vi "Actor Core.vi"(8 "error in":errorcluster, 11 "Rotation View in":refnum<class "Rotation View.lvclass">) -> (0 "error out":errorcluster, 3 "Actor out":refnum<class "Actor.lvclass">)   [LabVIEW 2020, in "Rotation View.lvlib" / "Rotation View.lvclass"]
doc: "(<B>Filename</B>: Actor Framework.lvlib:Actor.lvclass:Actor Core.vi)\n\nReceives messages to the actor, reacts to them, and initiates any error handling that may shut the actor down.\n\nDescendant classes may override this VI to append parallel tasks for the actor to complete while it handles messages. Overrides use the Call Parent Method node."
uses:
  Rotation View.lvclass
  C:/Program Files/National Instruments/LabVIEW 2020/vi.lib/ActorFramework/Actor/Actor.lvclass
  <vilib>/ActorFramework/Actor/Actor.lvclass
  Rotation View.lvclass/Rotation View.ctl
  <vilib>/ActorFramework/Actor/Actor.lvclass/Actor.ctl
  <vilib>/ActorFramework/Message Enqueuer/Message Enqueuer.lvclass/Message Enqueuer.ctl
  Rotation View Messages/Broadcast Preview Rotation Angle Msg/Broadcast Preview Rotation Angle Msg.lvclass/Broadcast Preview Rotation Angle Msg.ctl
  Rotation View Messages/Broadcast Rotation Angle Msg/Broadcast Rotation Angle Msg.lvclass/Broadcast Rotation Angle Msg.ctl
  <vilib>/ActorFrameworkMVC/View Controller/View Controller Messages/Remove Subpanel Msg/Remove Subpanel Msg.lvclass/Remove Subpanel Msg.ctl
  <vilib>/ActorFramework/Message Enqueuer/Init from Existing Queue.vi
  <vilib>/ActorFramework/Message Enqueuer/Enqueue.vi
  Rotation View Messages/Broadcast Preview Rotation Angle Msg/Broadcast Preview Rotation Angle Msg.lvclass
  C:/Program Files/National Instruments/LabVIEW 2020/vi.lib/ActorFramework/Message/Message.lvclass
  Rotation View Messages/Broadcast Rotation Angle Msg/Broadcast Rotation Angle Msg.lvclass
  Controllers/UI Controller/UI Controller Messages/Initialize Main View Msg/Initialize Main View Msg.lvclass
  <vilib>/ActorFrameworkMVC/View Controller/View Controller Messages/Remove Subpanel Msg/Remove Subpanel Msg.lvclass
  Rotation View Messages/Broadcast Cancel Rotation Msg/Broadcast Cancel Rotation Msg.lvclass
  <vilib>/ActorFramework/Message Priority Queue/Priority Enqueue.vi
  <vilib>/ActorFrameworkMVC/Abstract View/Abstract View/Abstract View.lvclass
  <vilib>/ActorFramework/Message Enqueuer/Message Enqueuer.lvclass
panel:
  in  "Set Button":bool
  in  "Close Button":bool
  in  "Rotation Angle Slider":dbl(slide) scale=-180.0..180.0
  # "Rotation angle (degree)"
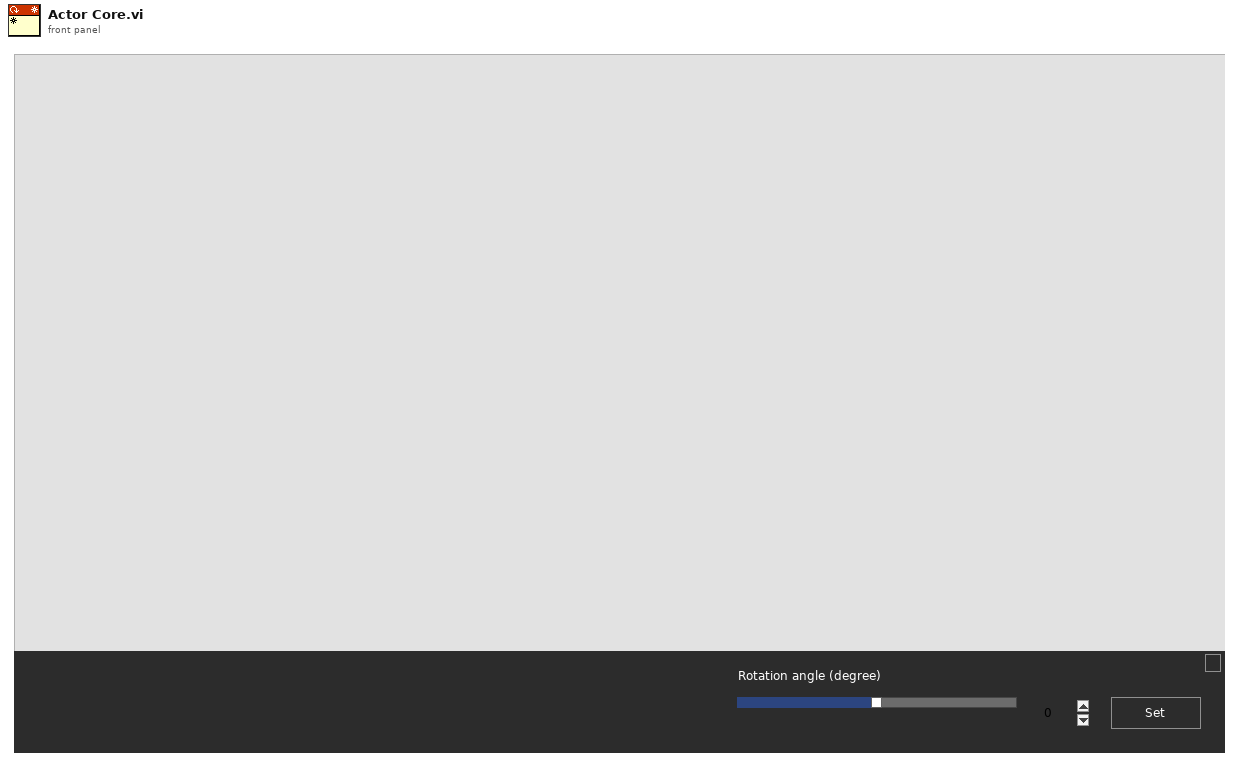
[diagram p1: front panel]
types:
  T1 = enum8{"Enabled", "Disabled", "Disabled and Grayed Out"}
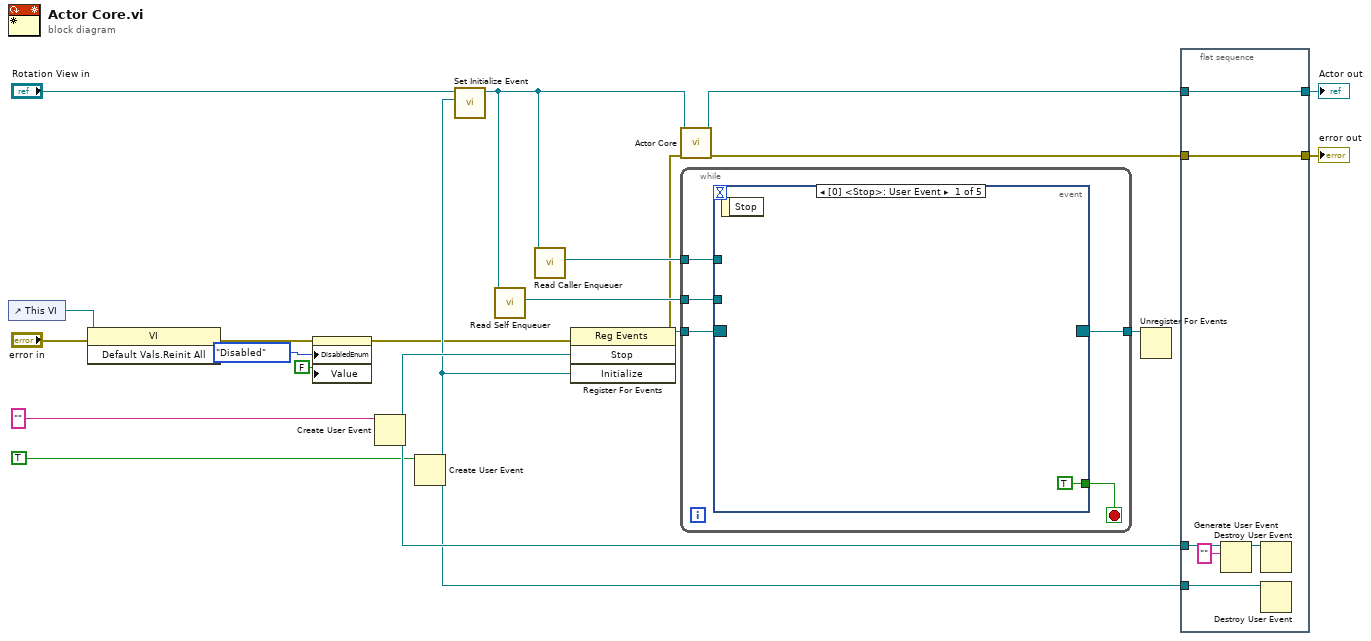
[diagram p0: block diagram]
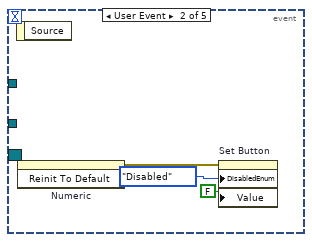
[diagram p2: hidden frame]
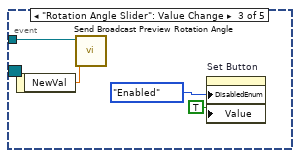
[diagram p3: hidden frame]
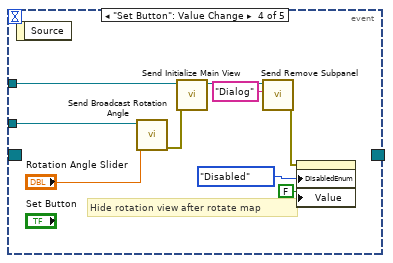
[diagram p4: hidden frame]
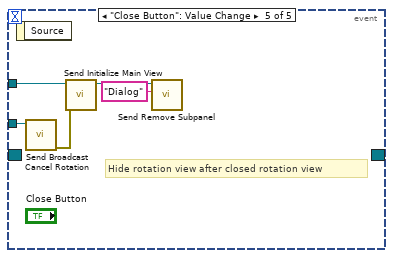
[diagram p5: hidden frame]
diagram:
  n1 = control-ref of="This VI"() -> (w14:refnum<vi>)
  n2 = invoke class="VI" method="Default Vals.Reinit All"(reference=w14, error in="error in") -> (error out=w3:errorcluster)  [unwired: 1 in, 2 out]
  n3 = property on="Set Button" class="Bool (strict)"(error in=w3, "DisabledEnum"=T1."Disabled" ("Disabled"), "Value"=FALSE ("Set Button")) -> (error out=w2:errorcluster)  [unwired: 1 in, 1 out]
  n4 = Create User Event(user event datatype="" ("Stop")) -> (user event=w15:refnum<user-event>)  [unwired: 1 in, 1 out]
  n5 = Create User Event(user event datatype=TRUE ("Initialize")) -> (user event=w7:refnum<user-event>)  [unwired: 1 in, 1 out]
  n6 = call "Set Initialize Event.vi"("Initialize Event"=w7, "Rotation View in"="Rotation View in") -> ("Rotation View out"=w1:refnum<class "Rotation View.lvclass">)  [unwired: 9 in]
  n7 = call <vilib>:"Read Self Enqueuer.vi"("Actor"=w1) -> ("Self Enqueuer"=w16:refnum<class "Message Enqueuer.lvclass">)  [unwired: 10 in]
  n8 = call <vilib>:"Read Caller Enqueuer.vi"("Actor"=w1) -> ("Caller Enqueuer"=w13:refnum<class "Message Enqueuer.lvclass">)  [unwired: 10 in]
  n9 = register-events(error in=w2, w15, w7) -> (reference out=w19:refnum<event-registration>, error out=w6:errorcluster)  [unwired: 1 in]
  n10 = call-parent "Actor Core.vi"("error in"=w6, "Abstract View in"=w1) -> ("error out"=w17:errorcluster, "Actor out"=w18:refnum<class "Actor.lvclass">)  [unwired: 8 in]
  n11 = while {
    tunnel: w19 -> [w26]
    tunnel: [w25] -> w20
    tunnel: w16 -> [w23]
    tunnel: w13 -> [w22]
    stop <- w24 stop-if-true
    n12 = event shown="[0] <Stop>: User Event" {
      selector: w26 -> [_ _ _ _ _]
      dyn-events: [_ _ _ _ _] -> w25
      timeout: _ -> [_ _ _ _ _]
      tunnel: [TRUE _ _ _ _] -> w24
      tunnel: w23 -> [_ _ w34 w43 w45]
      tunnel: w22 -> [_ _ _ w39 w48]
      event User Event {
        n13 = event-data() -> ()  [unwired: 1 in, 1 out]
      }
      event User Event {
        n14 = event-data() -> ()  [unwired: 1 in, 1 out]
        n15 = invoke on="Numeric" class="DigNum (strict)" method="Reinit To Default"() -> (error out=w28:errorcluster)  [unwired: 3 in, 2 out]
        n16 = property on="Set Button" class="Bool (strict)"(error in=w28, "DisabledEnum"=T1."Disabled" ("Disabled"), "Value"=FALSE ("Set Button")) -> ()  [unwired: 1 in, 2 out]
      }
      event "Rotation Angle Slider": Value Change {
        n17 = event-data() -> ("NewVal"=w33:dbl)  [unwired: 1 in]
        n18 = call "Send Broadcast Preview Rotation Angle.vi"("Rotation Preview Angle"=w33, "Message Enqueuer"=w34) -> ()  [unwired: 8 in, 2 out]
        n19 = property on="Set Button" class="Bool (strict)"("DisabledEnum"=T1."Enabled" ("Disabled"), "Value"=TRUE ("Set Button")) -> ()  [unwired: 2 in, 2 out]
      }
      event "Set Button": Value Change {
        # "Hide rotation view after rotate map"
        n20 = event-data() -> ()  [unwired: 1 in, 1 out]
        n21 = call "Send Broadcast Rotation Angle.vi"("Rotation Angle"="Rotation Angle Slider", "Message Enqueuer"=w43) -> ("error out"=w38:errorcluster)  [unwired: 8 in, 1 out]
        n22 = call "Send Initialize Main View.vi"("error in (no error)"=w38, "Message Enqueuer"=w39) -> ("Message Enqueuer out"=w41:refnum<class "Message Enqueuer.lvclass">)  [unwired: 8 in, 1 out]
        n23 = call <vilib>:"Send Remove Subpanel.vi"("Subpanel Name"="Dialog", "Message Enqueuer"=w41) -> ("error out"=w35:errorcluster)  [unwired: 8 in, 1 out]
        n24 = property on="Set Button" class="Bool (strict)"(error in=w35, "DisabledEnum"=T1."Disabled" ("Disabled"), "Value"=FALSE ("Set Button")) -> ()  [unwired: 1 in, 2 out]
      }
      event "Close Button": Value Change {
        # "Hide rotation view after closed rotation view"
        n25 = event-data() -> ()  [unwired: 1 in, 1 out]
        n26 = call "Send Broadcast Cancel Rotation.vi"("Message Enqueuer"=w45) -> ("error out"=w44:errorcluster)  [unwired: 9 in, 1 out]
        n27 = call "Send Initialize Main View.vi"("error in (no error)"=w44, "Message Enqueuer"=w48) -> ("Message Enqueuer out"=w47:refnum<class "Message Enqueuer.lvclass">)  [unwired: 8 in, 1 out]
        n28 = call <vilib>:"Send Remove Subpanel.vi"("Subpanel Name"="Dialog", "Message Enqueuer"=w47) -> ()  [unwired: 8 in, 2 out]
      }
    }
  }
  n29 = Unregister For Events(event registration refnum=w20) -> ()  [unwired: 1 in, 1 out]
  n30 = flat-sequence {
    tunnel: w15 -> [w53]
    tunnel: w18 -> [w51]
    tunnel: [w51] -> w10
    tunnel: [w50] -> w9
    tunnel: w17 -> [w50]
    tunnel: w7 -> [w49]
    frame #0 {
      n31 = Generate User Event(user event=w53, event data cluster="" ("event data")) -> (user event out=w54:refnum<user-event>)  [unwired: 2 in, 1 out]
      n32 = Destroy User Event(user event=w54) -> ()  [unwired: 1 in, 1 out]
      n33 = Destroy User Event(user event=w49) -> ()  [unwired: 1 in, 1 out]
    }
  }
  "error out" <- w9
  "Actor out" <- w10
